vi "TCP_Main.vi"() -> ()   [LabVIEW 2024]
uses:
  <vilib>/Platform/TimedLoop/XDataNode/timing_clust.ctl
  <vilib>/Platform/TimedLoop/XDataNode/nitl_modes.ctl
  <vilib>/Platform/TimedLoop/XDataNode/wakeup.ctl
  <vilib>/addons/Maxon Motor/EPOS2 CANopen/CANopen/sbCANopenBaseClass.lvclass
  <vilib>/platform/TimedLoop/XDataNode/XDataNode.xnode
  <vilib>/Platform/TimedLoop/XDataNode/XDNodeRunTimeDep.lvlib
panel:
  out "TCP Read Error":errorcluster
  out "goal_Tensions":dbl[](array[numeric])
  out "ResetPID":bool
  in  "Motor_index":i32[](array[numeric])=[3, 6, 9, 12, 2, 7, 8, 13, 4, 5, 10, 11, 1, 14]
  out "canERROR":errorcluster[][](array[cluster])
  in  "Control Mode":string="O"
  in  "TARE":bool
  in  "curr_Tensions":dbl[](array[numeric])
  out "DAQ Error":errorcluster
  out "Write Late?":bool
  out "Write Time [us]":i64
  in  "Tare_Tensions":dbl[](array[numeric])=[1.6875269817998764, 0.7228096971601798, 1.962272927280566, 2.6696462364433735, 2.7003690389898463, 3.088938448864716, 1.6430905755314908, 3.0754139877790347, 3.5546581214666455, 3.2737863413382597, 4.727265898547672, 2.6001067118162604, 1.980007529135911, 1.8614502099489874]
  in  "STOP CONTROLLER":bool
  # "\"Error\" codes:\n\n66 - Client Disconnected\n56 - TCP Read time out (every 1ms if no msg comes in)\n0 - packet received"
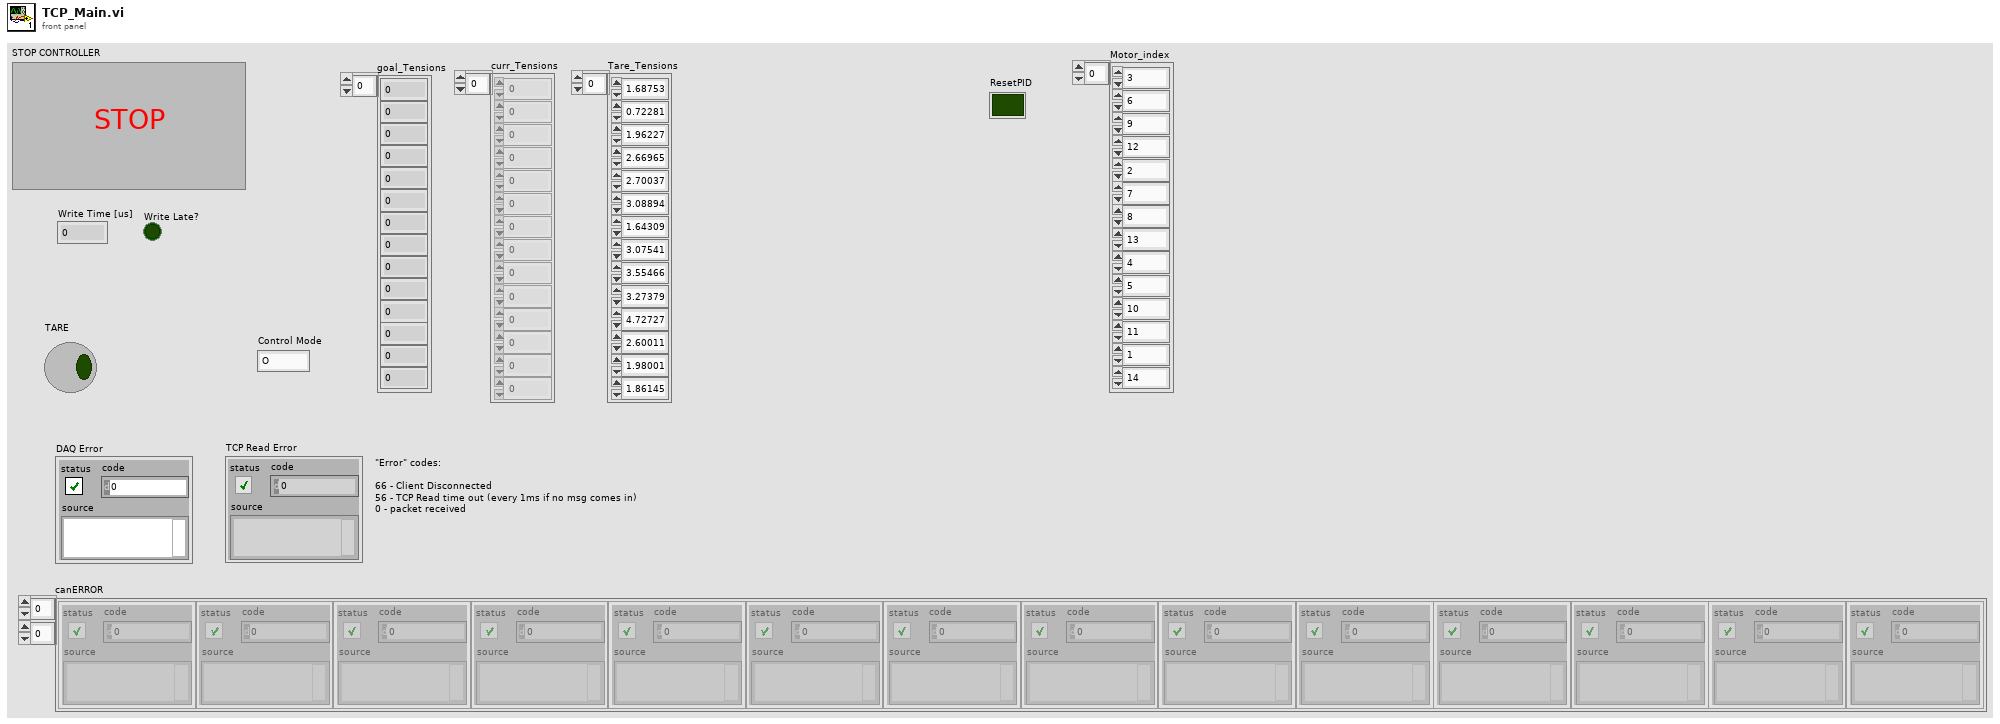
[diagram p1: front panel]
types:
  T1 = enum16{"Standard", "Buffered", "CRLF", "Immediate"}
  T2 = typedef "XDNodeRunTimeDep.lvlib/timing_clust.ctl" = cluster{"Expected End [f-1]":u64, "Actual End [f-1]":u64, "Finished Late? [f-1]":bool, "Expected End [i-1]":u64, "Actual End [i-1]":u64, "Finished Late? [i-1]":bool, "Expected Start [i]":u64, "Actual Start [i]":u64, "Expected Start [f]":u64, "Actual Start [f]":u64, "Source Name":string, "Structure Name":string, "Period":i64, "Deadline":i64, "Offset":i64, "Start":i64, "Priority":i32, "Timeout":i32, "Mode":T3, "Wakeup Reason":T4, "Error":errorcluster, "Source Type":string, "Secondary Source Type":string, "Global End Time":u64, "Global Start Time":u64, "Frame Duration":u64, "Iteration Duration":u64, "Assigned CPU":i32, "I/O Scan Engine Mode":u32}
  T3 = typedef "XDNodeRunTimeDep.lvlib/nitl_modes.ctl" = enum32{"No Change", "Process missed periods, maintain original phase", "Discard missed periods, maintain original phase", "Process missed periods, ignore original phase", "Discard missed periods, ignore original phase"}
  T4 = typedef "XDNodeRunTimeDep.lvlib/wakeup.ctl" = enum32{"Normal", "Aborted", "Asynchronous wakeup", "Timing source error", "Timed loop error", "Timeout"}
  T5 = cluster{"curr_Tensions":dbl[], "goal_Tensions":dbl[]}
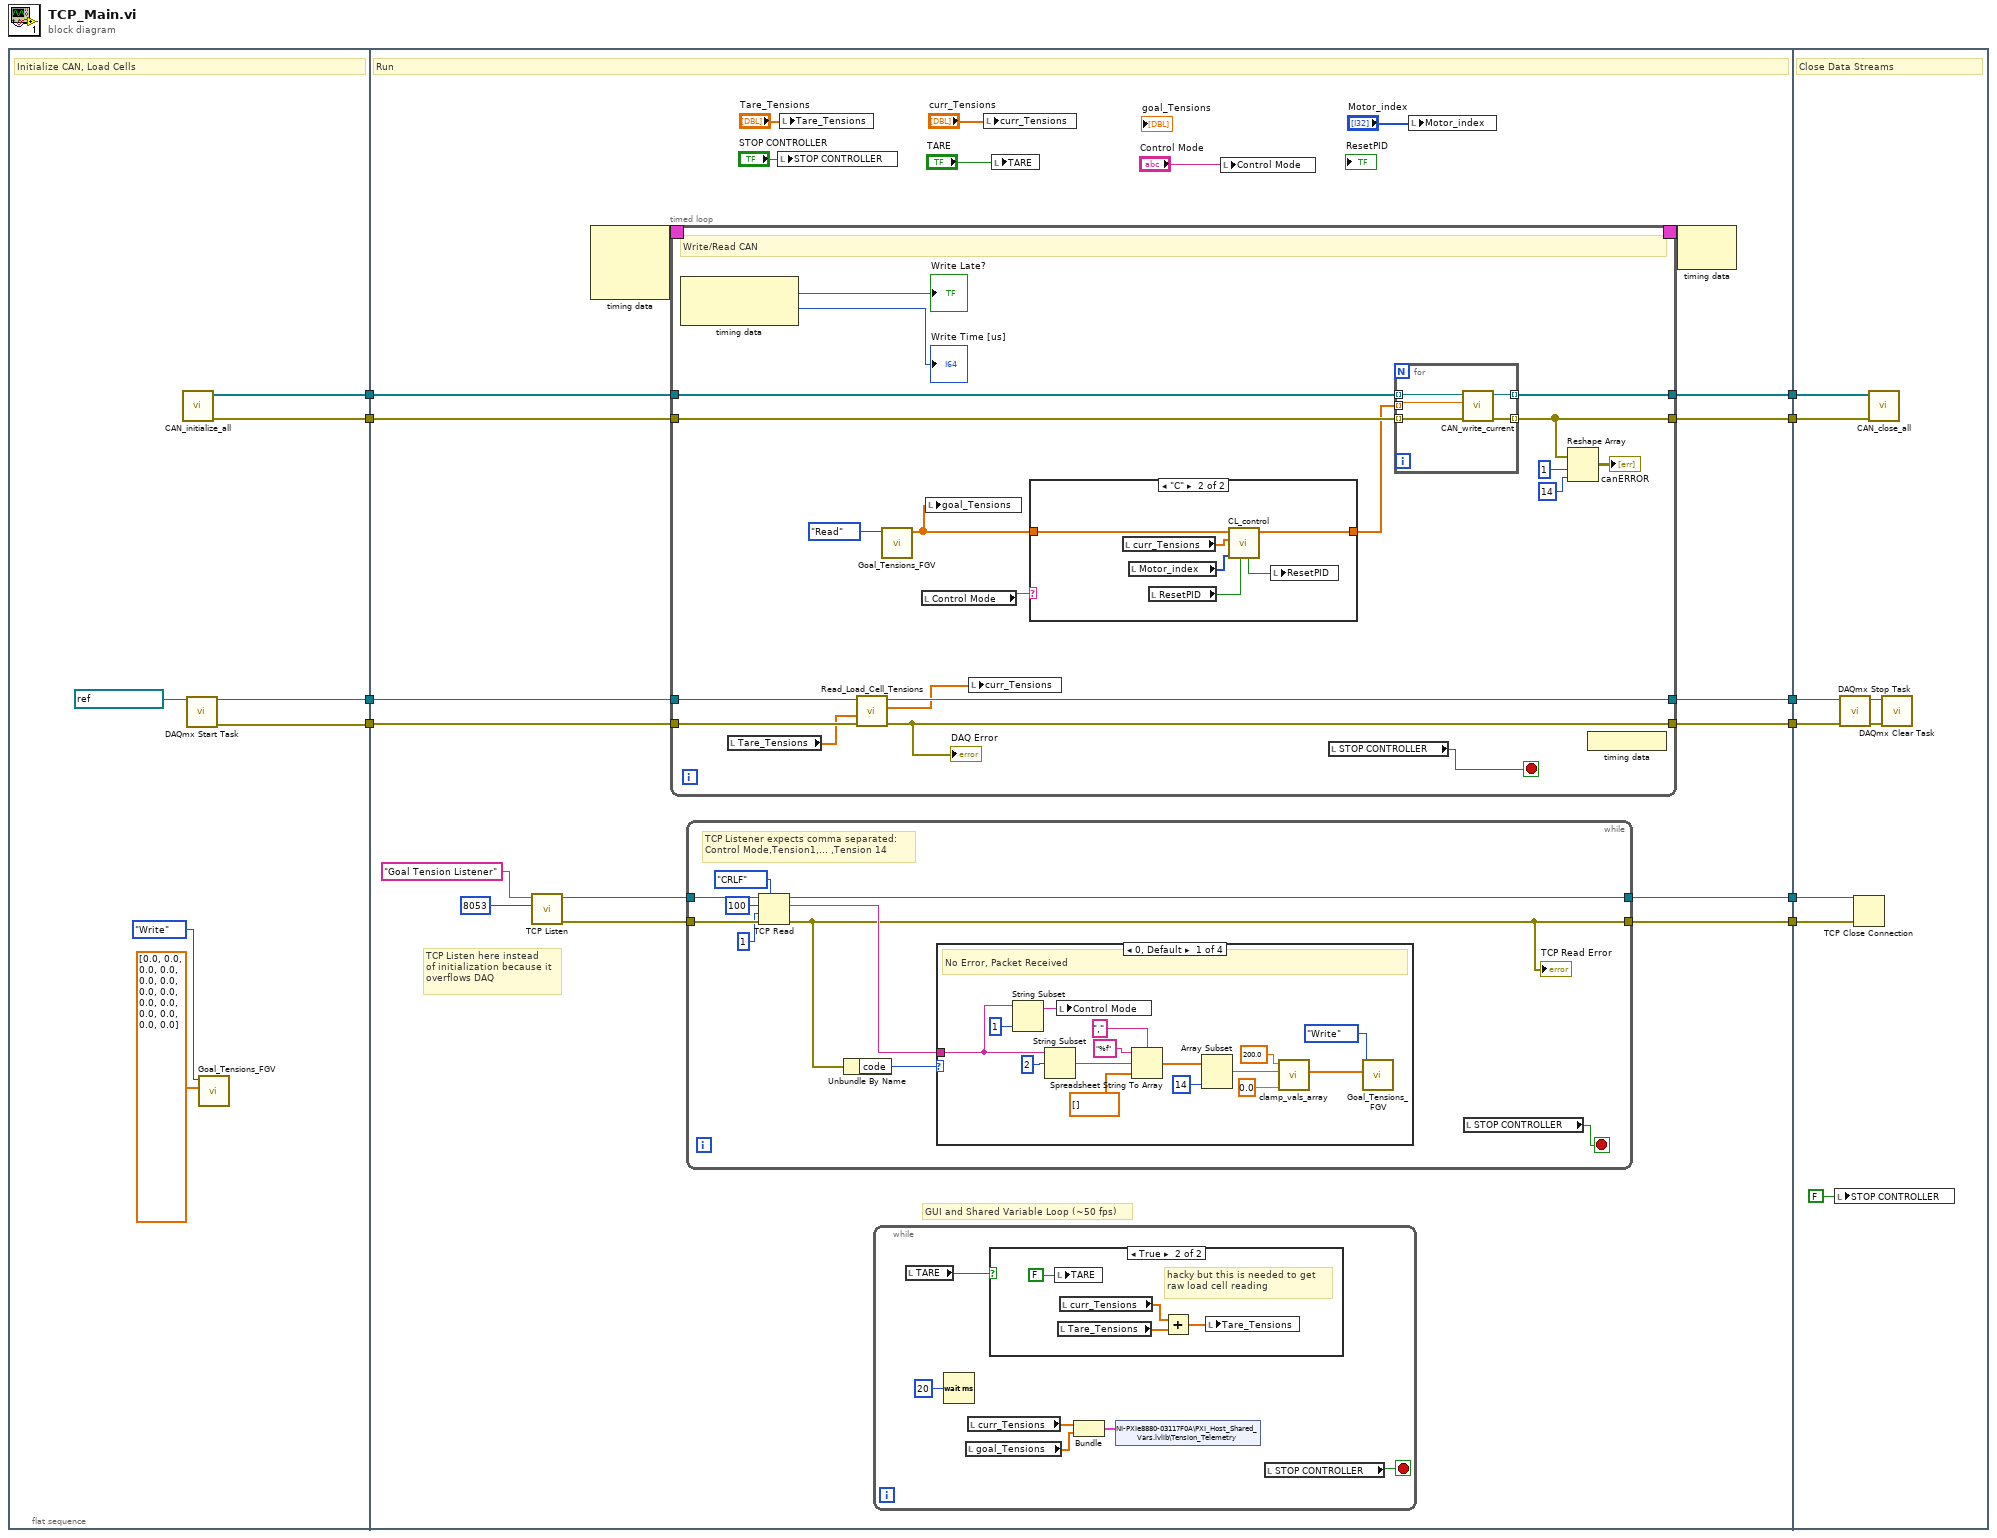
[diagram p0: block diagram]
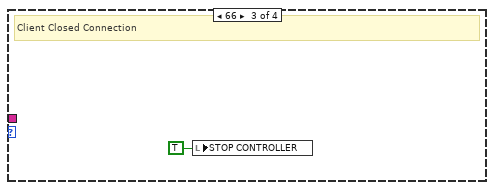
[diagram p3: hidden frame]
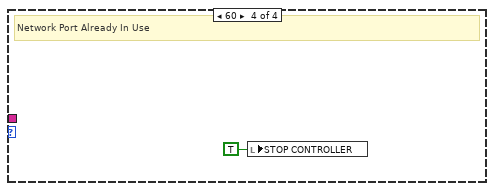
[diagram p4: hidden frame]
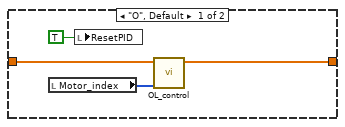
[diagram p6: hidden frame]
diagram:
  n1 = flat-sequence {
    tunnel: [w16] -> w10
    tunnel: [w17] -> w9
    tunnel: [w13] -> w6
    tunnel: [w14] -> w5
    tunnel: w10 -> [w37]
    tunnel: w9 -> [w36]
    tunnel: [w35] -> w8
    tunnel: [w34] -> w7
    tunnel: w6 -> [w32]
    tunnel: w5 -> [w31]
    tunnel: [w30] -> w4
    tunnel: [w29] -> w3
    tunnel: [w22] -> w2
    tunnel: [w23] -> w1
    tunnel: w8 -> [w126]
    tunnel: w7 -> [w125]
    tunnel: w4 -> [w122]
    tunnel: w3 -> [w121]
    tunnel: w2 -> [w119]
    tunnel: w1 -> [w118]
    frame #0 {
      # "Initialize CAN, Load Cells"
      n2 = call "CAN_initialize_all.vi"() -> ("Array of Canopen Sessions"=w17:refnum<class "sbCANopenBaseClass.lvclass">[], "Array of Error out's"=w16:errorcluster[])  [unwired: 5 in]
      n3 = call <vilib>:"DAQmx Start Task.vi"("task/channels in"=refnum<k21> "SCI_TenSen") -> ("task out"=w13:refnum<k21>, "error out"=w14:errorcluster)  [unwired: 13 in]
      n4 = call "Goal_Tensions_FGV.vi"("Write Goal Tension"=dbl[] [0.0, 0.0, 0.0, 0.0, 0.0, 0.0, 0.0, 0.0, 0.0, 0.0, 0.0, 0.0, 0.0, 0.0], "Operation"=enum16{"Write", "Read"}."Write") -> ()  [unwired: 9 in, 1 out]
    }
    frame #1 {
      # "TCP Listen here instead\nof initialization because it\noverflows DAQ"
      # "GUI and Shared Variable Loop (~50 fps)"
      # "Run"
      n5 = call <vilib>:"TCP Listen.vi"("port"=u16 8053, "service name"="Goal Tension Listener") -> ("error out"=w19:errorcluster, "connection ID"=w18:refnum<k5>)  [unwired: 5 in, 3 out]
      n6 = node-c288() -> (w39:T2)  [unwired: 3 in]
      n7 = timed-loop {
        tunnel: w37 -> [w88]
        tunnel: [w80] -> w35
        timing: w39 -> [_]
        timing-out: [_] -> w38
        tunnel: w36 -> [w89]
        tunnel: [w93] -> w34
        tunnel: w32 -> [w92]
        tunnel: w31 -> [w91]
        tunnel: [w90] -> w30
        tunnel: [w87] -> w29
        stop <- w94 stop-if-true
        # "Write/Read CAN"
        n8 = node-c288() -> (→"Write Late?":bool, →"Write Time [us]":i64)  [unwired: 1 in]
        n9 = local read "Tare_Tensions"() -> (w86:dbl[])
        n10 = call "Read_Load_Cell_Tensions.vi"("error in (no error)"=w91, "Tare Tension"=w86, "Refnum in"=w92) -> ("error out"=w87:errorcluster, "Measured Cable Tensions"=w84:dbl[], "Refnum out"=w90:refnum<k21>)  [unwired: 4 in]
        "DAQ Error" <- w87
        n11 = call "Goal_Tensions_FGV.vi"("Operation"=enum16{"Write", "Read"}."Read") -> ("Read Goal Tension"=w78:dbl[])  [unwired: 10 in]
        n12 = local read "Control Mode"() -> (w85:string)
        n13 = local write "goal_Tensions"(w78) -> ()
        n14 = local write "curr_Tensions"(w84) -> ()
        n15 = case shown="\"C\"" w85 {
          tunnel: [w100 w106] -> w83
          tunnel: w78 -> [w97 w101]
          frame "O", Default {
            n16 = local read "Motor_index"() -> (w99:i32[])
            n17 = local write "ResetPID"(TRUE) -> ()
            n18 = call "OL_control.vi"("Motor_index"=w99, "goal_Tensions"=w97) -> ("can_Current"=w100:dbl[])  [unwired: 9 in]
          }
          frame "C" {
            n19 = local read "curr_Tensions"() -> (w102:dbl[])
            n20 = local read "Motor_index"() -> (w105:i32[])
            n21 = local read "ResetPID"() -> (w104:bool)
            n22 = call "CL_control.vi"("ResetPID"=w104, "Motor_index"=w105, "curr_Tensions"=w102, "goal_Tensions"=w101) -> ("can_Current"=w106:dbl[], "Reset PID (output)"=w103:bool)  [unwired: 6 in]
            n23 = local write "ResetPID"(w103) -> ()
          }
        }
        n24 = local read "STOP CONTROLLER"() -> (w94:bool)
        n25 = for {
          tunnel: [w108] -> w93 mode=indexing
          tunnel: [w109] -> w80 mode=indexing
          tunnel: w89 -> [w111] mode=indexing
          tunnel: w88 -> [w110] mode=indexing
          tunnel: w83 -> [w107] mode=indexing
          n26 = call "CAN_write_current.vi"("error in"=w110, "Current Command [mA]"=w107, "CANopen Session In"=w111) -> ("error out"=w109:errorcluster, "CANopen Session Out"=w108:refnum<class "sbCANopenBaseClass.lvclass">)  [unwired: 7 in]
        }
        n27 = Reshape Array(w80, 1 ("dimension size"), 14 ("dimension size")) -> (→"canERROR":errorcluster[][])
        n28 = node-c288() -> ()  [unwired: 1 out]
      }
      n29 = while {
        tunnel: [w41] -> w22
        tunnel: [w49] -> w23
        tunnel: w19 -> [w47]
        tunnel: w18 -> [w46]
        stop <- w43 stop-if-true
        # "TCP Listener expects comma separated:\nControl Mode,Tension1,... ,Tension 14"
        n30 = TCP Read(connection ID=w46, bytes to read=100, error in (no error)=w47, 7:T1."CRLF" ("mode (standard)"), 9:1 ("timeout ms (25000)")) -> (connection ID out=w49:refnum<k5>, data out=w48:string, error out=w41:errorcluster)
        "TCP Read Error" <- w41
        n31 = Unbundle By Name(w41) -> ("code"=w42:i32)
        n32 = case shown="0, Default" w42 {
          tunnel: w48 -> [w62 _ _ _]
          frame 0, Default {
            # "No Error, Packet Received"
            n33 = String Subset(string=w62, length (rest)=1 ("length (rest)")) -> (substring=w63:string)  [unwired: 1 in]
            n34 = String Subset(string=w62, offset (0)=2) -> (substring=w60:string)  [unwired: 1 in]
            n35 = local write "Control Mode"(w63) -> ()
            n36 = Spreadsheet String To Array(delimiter (Tab)=",", format string="%f", spreadsheet string=w60, array type (2D Dbl)=dbl[] []) -> (array=w55:dbl[])
            n37 = Array Subset(array=w55, length=14) -> (w52:dbl[])  [unwired: 1 in]
            n38 = call "clamp_vals_array.vi"("Min Val"=0.0, "Input Array"=w52, "Max Val"=200.0) -> ("Output Array"=w51:dbl[])  [unwired: 8 in]
            n39 = call "Goal_Tensions_FGV.vi"("Write Goal Tension"=w51, "Operation"=enum16{"Write", "Read"}."Write") -> ()  [unwired: 9 in, 1 out]
          }
          frame 56 {
            # "continue"
            # "Time out Error"
          }
          frame 66 {
            # "Client Closed Connection"
            n40 = local write "STOP CONTROLLER"(TRUE ("STOP CONTROLLER")) -> ()
          }
          frame 60 {
            # "Network Port Already In Use"
            n41 = local write "STOP CONTROLLER"(TRUE ("STOP CONTROLLER")) -> ()
          }
        }
        n42 = local read "STOP CONTROLLER"() -> (w43:bool)
      }
      n43 = local write "STOP CONTROLLER"("STOP CONTROLLER") -> ()
      n44 = local write "Tare_Tensions"("Tare_Tensions") -> ()
      n45 = while {
        stop <- w72 stop-if-true
        n46 = local read "TARE"() -> (w71:bool)
        n47 = Wait (ms)(milliseconds to wait=u32 20) -> ()  [unwired: 1 out]
        n48 = local read "goal_Tensions"() -> (w67:dbl[])
        n49 = local read "curr_Tensions"() -> (w70:dbl[])
        n50 = case shown="True" w71 {
          frame False {
          }
          frame True {
            # "hacky but this is needed to get \nraw load cell reading"
            n51 = local write "TARE"(FALSE ("TARE")) -> ()
            n52 = local read "Tare_Tensions"() -> (w74:dbl[])
            n53 = local read "curr_Tensions"() -> (w75:dbl[])
            n54 = Add(x=w75, y=w74) -> (x+y=w76:dbl[])
            n55 = local write "Tare_Tensions"(w76) -> ()
          }
        }
        n56 = Bundle("curr_Tensions"=w70, "goal_Tensions"=w67) -> (w69:T5)  [unwired: 1 in]
        n57 = shared-variable "NI-PXIe8880-03117F0A\\PXI_Host_Shared_Vars.lvlib\\Tension_Telemetry"(w69) -> ()  [unwired: 1 in, 1 out]
        n58 = local read "STOP CONTROLLER"() -> (w72:bool)
      }
      n59 = local write "curr_Tensions"("curr_Tensions") -> ()
      n60 = local write "TARE"("TARE") -> ()
      n61 = local write "Control Mode"("Control Mode") -> ()
      n62 = local write "Motor_index"("Motor_index") -> ()
      n63 = node-c288(w38) -> ()  [unwired: 1 out]
    }
    frame #2 {
      # "Close Data Streams"
      n64 = local write "STOP CONTROLLER"(FALSE ("STOP CONTROLLER")) -> ()
      n65 = call <vilib>:"DAQmx Stop Task.vi"("task/channels in"=w122, "error in"=w121) -> ("task out"=w123:refnum<k21>, "error out"=w124:errorcluster)  [unwired: 12 in]
      n66 = TCP Close Connection(connection ID=w118, error in (no error)=w119) -> ()  [unwired: 1 in, 2 out]
      n67 = call "CAN_close_all.vi"("Input Error out array"=w126, "Input CANopen Sessions array"=w125) -> ()  [unwired: 10 in]
      n68 = call <vilib>:"DAQmx Clear Task.vi"("task in"=w123, "error in"=w124) -> ()  [unwired: 13 in, 1 out]
    }
  }
